vi "Configure Averaging.vi"(8 "error in (no error)":errorcluster, 9 "Enable Averge Mode  (on:T)":bool=TRUE, 10 "Average count (1)":i16=1 min=1 max=256 step=1, 11 "VISA resource name":refnum<visa-resource-name>) -> (0 "error out":errorcluster, 3 "VISA resource name out":refnum<visa-resource-name>)   [LabVIEW 2016, in "Agilent 4263X.lvlib"]
doc: "This VI configures the averaging mode of the instrument."
uses:
  <instrlib>/Agilent 4263X/Agilent 4263X.lvlib
panel:
  # "on\noff"
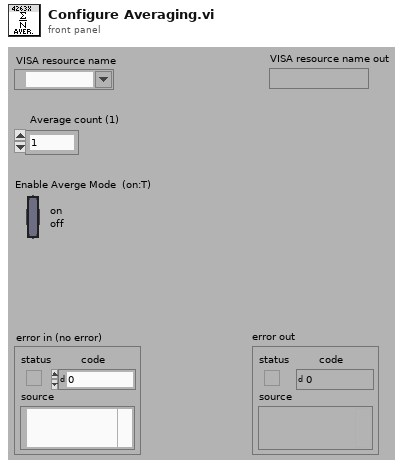
[diagram p1: front panel]
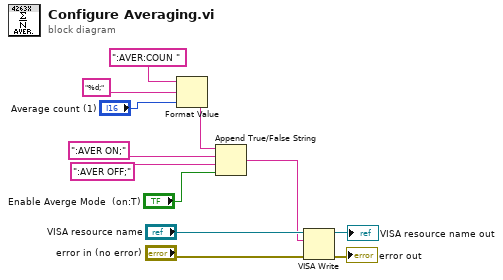
[diagram p0: block diagram]
diagram:
  n1 = Format Value(string ("")=":AVER:COUN ", format string="%d;", value (0)="Average count (1)") -> (output string=w5:string)
  n2 = Append True/False String(1:"Enable Averge Mode  (on:T)", 2:":AVER OFF;", 3:":AVER ON;", 4:w5) -> (0:w1:string)
  n3 = VISA Write(VISA resource name="VISA resource name", write buffer=w1, error in (no error)="error in (no error)") -> (VISA resource name out=→"VISA resource name out":refnum<visa-resource-name>, error out=→"error out":errorcluster)  [unwired: 1 out]
